vi "TRPES_save_xml_log.vi"(3 "Error In":errorcluster, 4 "XMLcluster-Jet":T1, 5 "XML File Path":path, 6 "Write XML":bool) -> (0 "Error Out":errorcluster, 2 "XML String Out":string)   [LabVIEW 2020]
uses:
  Type defs/XML_info_TRPES.ctl
  <vilib>/NI/GXML/GXML.lvlib
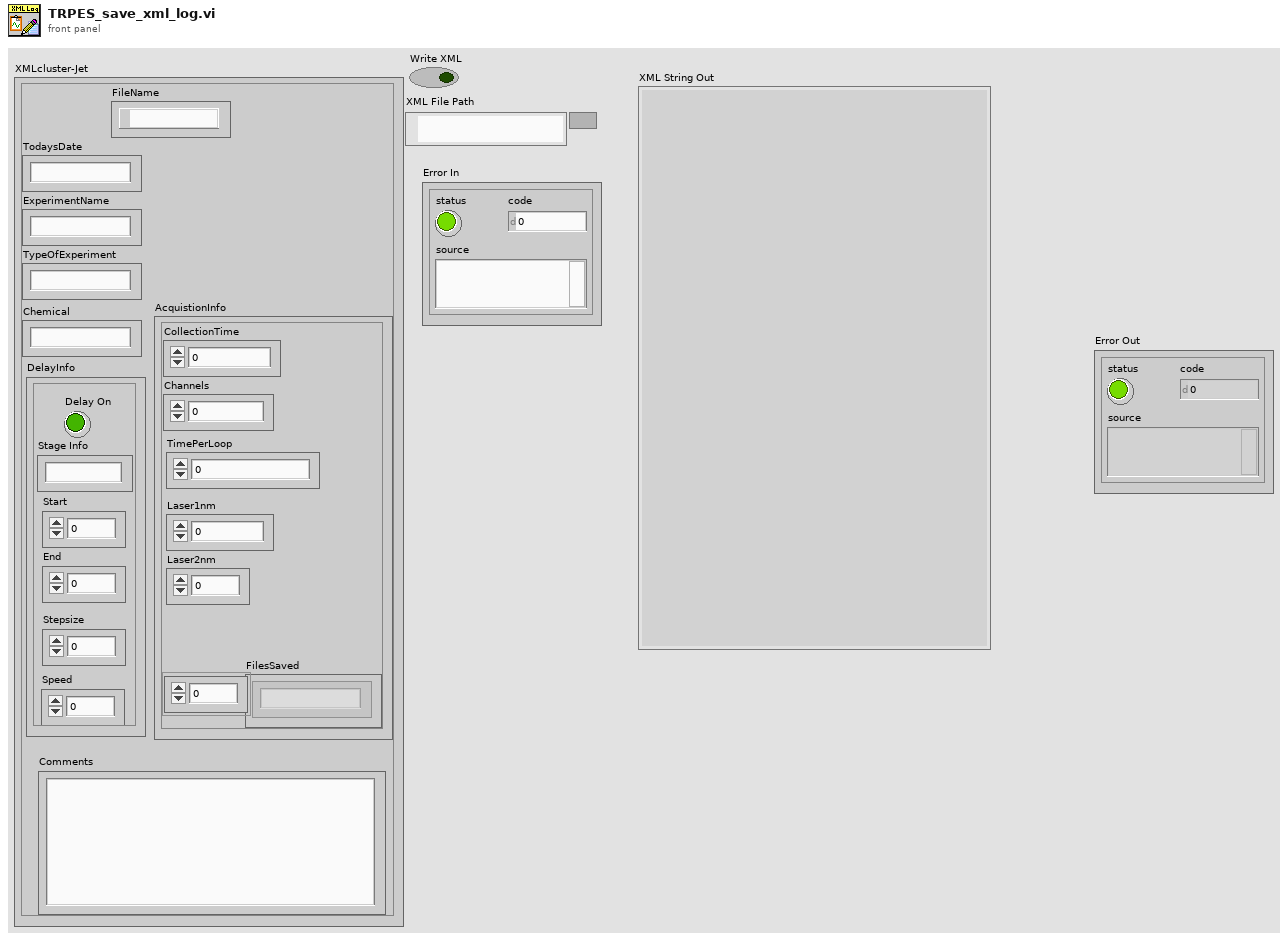
[diagram p1: front panel]
types:
  T1 = typedef "XML_info_TRPES.ctl" = cluster{"FileName":path, "TodaysDate":string, "ExperimentName":string, "TypeOfExperiment":string, "AcquistionInfo":cluster{"CollectionTime":dbl, "Channels":dbl, "TimePerLoop":dbl, "FilesSaved":string[], "Laser1nm":dbl, "Laser2nm":dbl}, "Chemical":string, "DelayInfo":cluster{"Start":dbl, "End":dbl, "Stepsize":dbl, "Speed":dbl, "Stage Info":string, "Delay On":bool}, "Comments":string}
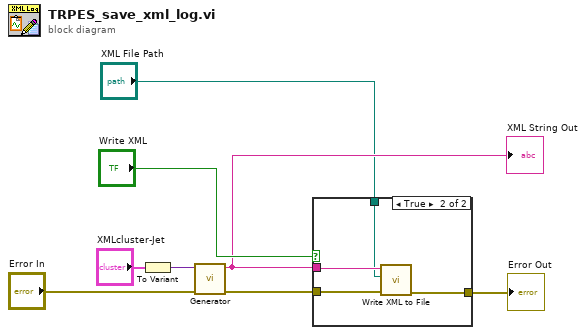
[diagram p0: block diagram]
diagram:
  n1 = To Variant(anything="XMLcluster-Jet") -> (Variant=w7:variant)
  n2 = call <vilib>:"Generator.vi"("error in"="Error In", "Variant"=w7) -> ("error out"=w4:errorcluster, "XML String Out"=w3:string)  [unwired: 8 in]
  "XML String Out" <- w3
  n3 = case shown="True" "Write XML" {
    tunnel: w4 -> [w9 w13]
    tunnel: w3 -> [_ w12]
    tunnel: [w9 w11] -> w2
    tunnel: "XML File Path" -> [_ w10]
    frame False {
    }
    frame True {
      n4 = call <vilib>:"Write XML to File.vi"("error in"=w13, "XML File Path"=w10, "XML Input"=w12) -> ("error out"=w11:errorcluster)  [unwired: 8 in]
    }
  }
  "Error Out" <- w2
